vi "TEST - Conditional Auto-Indexing Tunnel.vi"(8 "error in (no error)":errorcluster) -> (0 "error out":errorcluster, 2 "Pass?":bool=TRUE)   [LabVIEW 2009]
doc: "This VI template can be used for the functional testing of VIs; this implementation includes handling for the testing of polymorphic VIs, and the polymorphic elements should be removed if not needed.\n\nCoded by Douglas A. Femec, January 24, 2006.\n\nCopyright (c) 2005-2006 MKS Instruments, Inc.\nAll rights reserved."
uses:
  TEST - Conditional Auto-Indexing Tunnel - Inputs.ctl
  Polymorphizer+ Data Type.ctl
  TEST - Conditional Auto-Indexing Tunnel - Outputs.ctl
  source/library/Conditional Auto-Indexing Tunnel/Conditional Auto-Indexing Tunnel (EXT).vi
  source/library/Conditional Auto-Indexing Tunnel/Conditional Auto-Indexing Tunnel (U64).vi
  source/library/Conditional Auto-Indexing Tunnel/Conditional Auto-Indexing Tunnel (I64).vi
  source/library/Conditional Auto-Indexing Tunnel/Conditional Auto-Indexing Tunnel (DBL).vi
  source/library/Conditional Auto-Indexing Tunnel/Conditional Auto-Indexing Tunnel (SGL).vi
  source/library/Conditional Auto-Indexing Tunnel/Conditional Auto-Indexing Tunnel (I32).vi
  source/library/Conditional Auto-Indexing Tunnel/Conditional Auto-Indexing Tunnel (I16).vi
  source/library/Conditional Auto-Indexing Tunnel/Conditional Auto-Indexing Tunnel (I8).vi
  source/library/Conditional Auto-Indexing Tunnel/Conditional Auto-Indexing Tunnel (U32).vi
  source/library/Conditional Auto-Indexing Tunnel/Conditional Auto-Indexing Tunnel (LVObject).vi
  source/library/Conditional Auto-Indexing Tunnel/Conditional Auto-Indexing Tunnel (U16).vi
  source/library/Conditional Auto-Indexing Tunnel/Conditional Auto-Indexing Tunnel (U8).vi
  source/library/Conditional Auto-Indexing Tunnel/Conditional Auto-Indexing Tunnel (CXT).vi
  source/library/Conditional Auto-Indexing Tunnel/Conditional Auto-Indexing Tunnel (CDB).vi
  source/library/Conditional Auto-Indexing Tunnel/Conditional Auto-Indexing Tunnel (CSG).vi
  source/library/Conditional Auto-Indexing Tunnel/Conditional Auto-Indexing Tunnel (Bool).vi
  source/library/Conditional Auto-Indexing Tunnel/Conditional Auto-Indexing Tunnel (String).vi
  source/library/Conditional Auto-Indexing Tunnel/Conditional Auto-Indexing Tunnel (Path).vi
  source/library/Conditional Auto-Indexing Tunnel/Conditional Auto-Indexing Tunnel (Variant).vi
  source/library/Conditional Auto-Indexing Tunnel/Conditional Auto-Indexing Tunnel (CTL-REF).vi
  source/library/Conditional Auto-Indexing Tunnel/Conditional Auto-Indexing Tunnel (GEN-REF).vi
  source/library/Conditional Auto-Indexing Tunnel/Conditional Auto-Indexing Tunnel (GObj-REF).vi
  source/library/Conditional Auto-Indexing Tunnel/Conditional Auto-Indexing Tunnel (VI-REF).vi
  TestClass/TestClass.lvclass
panel:
  in  "VI Refnum":refnum<vi>
  in  "GObj Refnum":refnum<vi>
  in  "Gen Refnum":refnum<vi>
  in  "Ctl Refnum":refnum<vi>
  out "Generated Outputs":T1[][](array[typedef]) {"Filtered Array Out" format="%.2f"}
  in  "Expected Outputs":T1[](array[typedef])=[{"Description"="Expect empty array", "Filtered Array Out"=[]}, {"Description"="Expect no elements kept", "Filtered Array Out"=[]}, {"Description"="Expect some elements kept", "Filtered Array Out"=[0.0, 0.0]}, {"Description"="Expect all elements kept", "Filtered Array Out"=[0.0, 1.0, 0.0, 1.0]}] {"Filtered Array Out" format="%.2f"}
  in  "Inputs":T2[](array[typedef])=[{"Description"="Empty arrays", "Data Types to Test"=[enum."EXT", enum."DBL", enum."SGL", enum."I32", enum."I16", enum."I8", enum."U32", enum."U16", enum."U8", enum."CXT", enum."CDB", enum."CSG", enum."Boolean", enum."String", enum."Path", enum."Variant", enum."CTL-REF", enum."GEN-REF", enum."GObj-REF", enum."VI-REF", enum."I64", enum."U64", enum."LabVIEW Object"], "Elements to keep"=[], "Array In"=[]}, {"Description"="No elements to keep", "Data Types to Test"=[enum."EXT", enum."DBL", enum."SGL", enum."I32", enum."I16", enum."I8", enum."U32", enum."U16", enum."U8", enum."CXT", enum."CDB", enum."CSG", enum."Boolean", enum."String", enum."Path", enum."Variant", enum."CTL-REF", enum."GEN-REF", enum."GObj-REF", enum."VI-REF", enum."I64", enum."U64", enum."LabVIEW Object"], "Elements to keep"=[FALSE, FALSE, FALSE, FALSE], "Array In"=[0.0, 0.0, 0.0, 0.0]}, {"Description"="Keep some elements", "Data Types to Test"=[enum."EXT", enum."DBL", enum."SGL", enum."I32", enum."I16", enum."I8", enum."U32", enum."U16", enum."U8", enum."CXT", enum."CDB", enum."CSG", enum."Boolean", enum."String", enum."Path", enum."Variant", enum."CTL-REF", enum."GEN-REF", enum."GObj-REF", enum."VI-REF", enum."I64", enum."U64", enum."LabVIEW Object"], "Elements to keep"=[TRUE, FALSE, TRUE, FALSE], "Array In"=[0.0, 1.0, 0.0, 1.0]}, {"Description"="Keep all elements", "Data Types to Test"=[enum."EXT", enum."DBL", enum."SGL", enum."I32", enum."I16", enum."I8", enum."U32", enum."U16", enum."U8", enum."CXT", enum."CDB", enum."CSG", enum."Boolean", enum."String", enum."Path", enum."Variant", enum."CTL-REF", enum."GEN-REF", enum."GObj-REF", enum."VI-REF", enum."I64", enum."U64", enum."LabVIEW Object"], "Elements to keep"=[TRUE, TRUE, TRUE, TRUE], "Array In"=[0.0, 1.0, 0.0, 1.0]}] {"Array In" format="%.2f"}
  # "Copyright (c) 2005-2006 MKS Instruments, Inc.\nAll rights reserved."
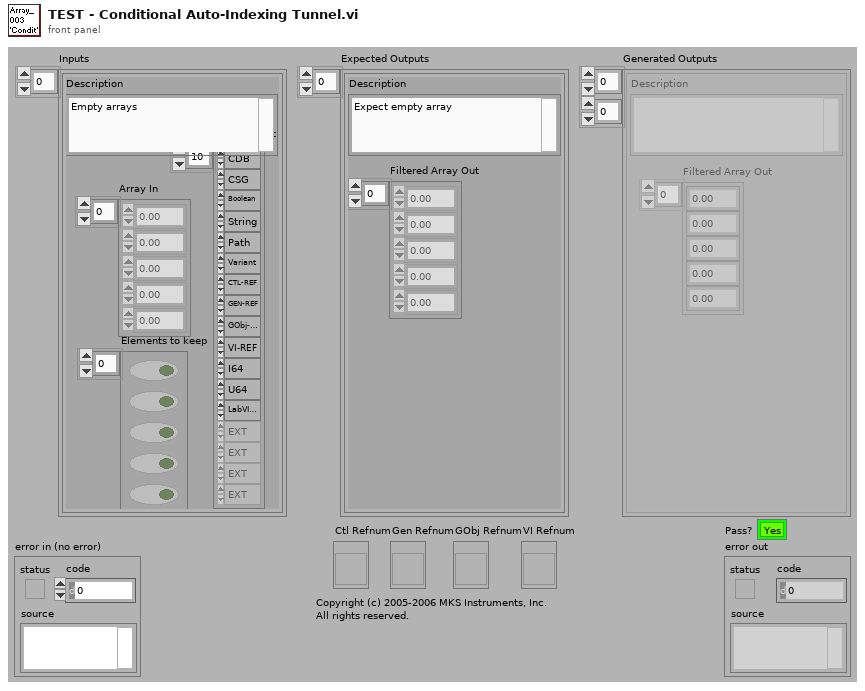
[diagram p1: front panel]
types:
  T1 = typedef "TEST - Conditional Auto-Indexing Tunnel - Outputs.ctl" = cluster{"Description":string, "Filtered Array Out":sgl[]}
  T2 = typedef "TEST - Conditional Auto-Indexing Tunnel - Inputs.ctl" = cluster{"Description":string, "Data Types to Test":T3[], "Elements to keep":bool[], "Array In":sgl[]}
  T3 = typedef "Polymorphizer+ Data Type.ctl" = enum16{"EXT", "DBL", "SGL", "I32", "I16", "I8", "U32", "U16", "U8", "CXT", "CDB", "CSG", "Boolean", "String", "Path", "Variant", "CTL-REF", "GEN-REF", "GObj-REF", "VI-REF", "ENUM", "ERR", "FILE-REF", "MENU-REF", "MENU-RING", "PICT-RING", "TXT&PICT-RING", "TXT-RING", "I64", "U64", "LabVIEW Object"}
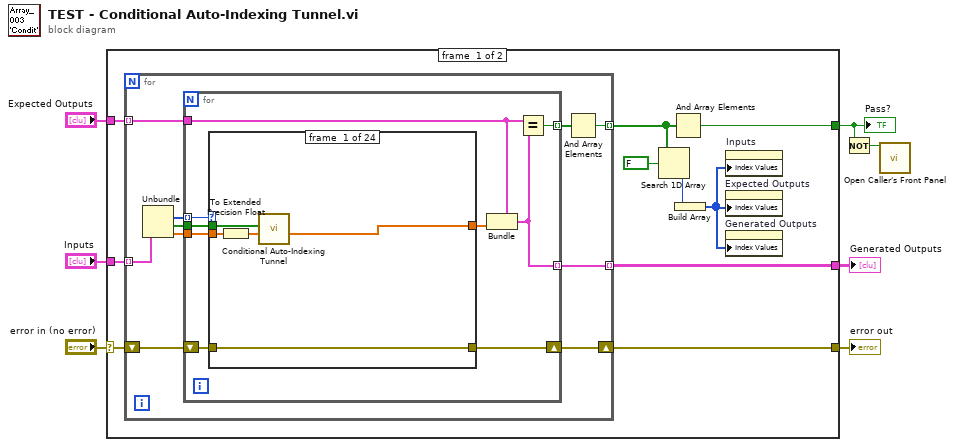
[diagram p0: block diagram]
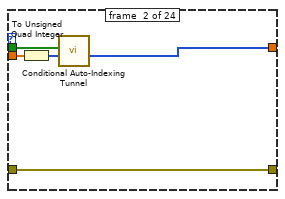
[diagram p2: hidden frame]
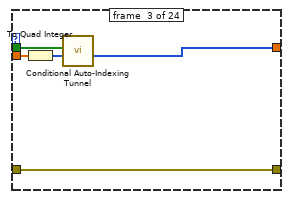
[diagram p3: hidden frame]
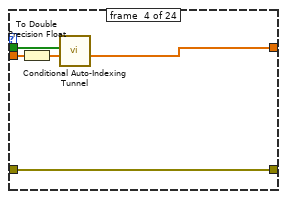
[diagram p4: hidden frame]
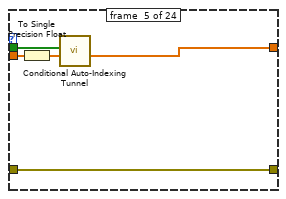
[diagram p5: hidden frame]
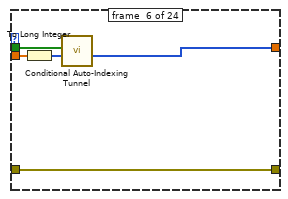
[diagram p6: hidden frame]
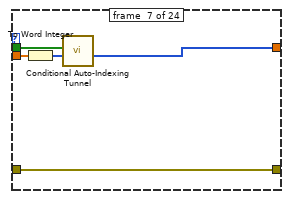
[diagram p7: hidden frame]
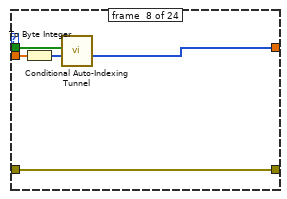
[diagram p8: hidden frame]
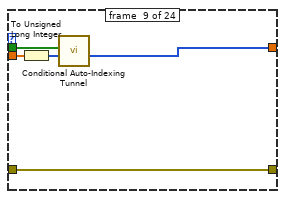
[diagram p9: hidden frame]
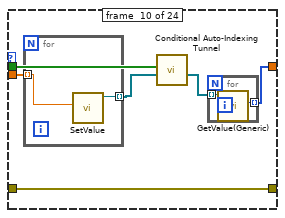
[diagram p10: hidden frame]
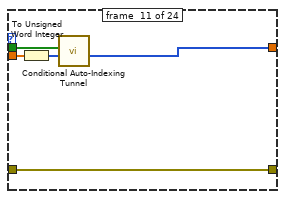
[diagram p11: hidden frame]
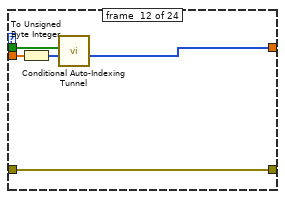
[diagram p12: hidden frame]
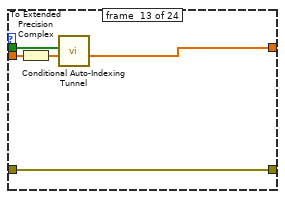
[diagram p13: hidden frame]
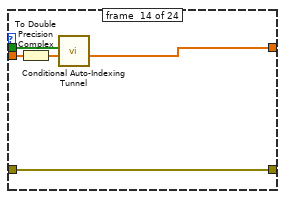
[diagram p14: hidden frame]
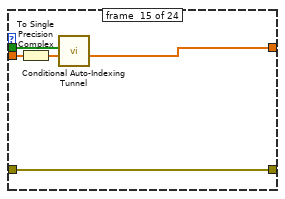
[diagram p15: hidden frame]
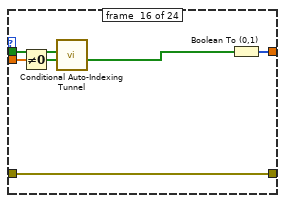
[diagram p16: hidden frame]
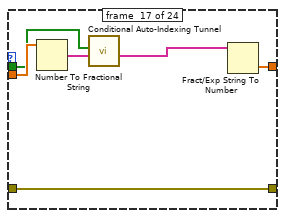
[diagram p17: hidden frame]
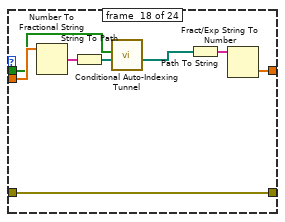
[diagram p18: hidden frame]
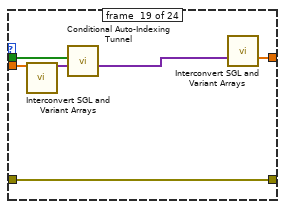
[diagram p19: hidden frame]
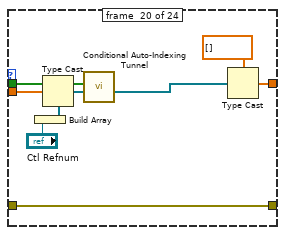
[diagram p20: hidden frame]
diagram:
  n1 = case shown="No Error" "error in (no error)" {
    selector: "error in (no error)" -> [w16 w181]
    tunnel: [w17 w181] -> w6
    tunnel: "Expected Outputs" -> [w14 _]
    tunnel: "Inputs" -> [w15 _]
    tunnel: [w13 _] -> w3
    tunnel: [w12 _] -> w1
    frame #0 {
      n2 = for {
        shift-right: [w22] -> w17
        shift-left: w16 -> [w23]
        tunnel: w15 -> [w24] mode=indexing
        tunnel: w14 -> [w27] mode=indexing
        tunnel: [w26] -> w13 mode=indexing
        tunnel: [w21] -> w11 mode=indexing
        n3 = Unbundle(w24) -> ("Data Types to Test"=w20:T3[], "Elements to keep"=w18:bool[], "Array In"=w19:sgl[])  [unwired: 1 out]
        n4 = for {
          tunnel: w27 -> [w36]
          tunnel: [w34] -> w26 mode=indexing
          tunnel: [w35] -> w25 mode=indexing
          shift-right: [w29] -> w22
          shift-left: w23 -> [w30]
          tunnel: w20 -> [w31] mode=indexing
          tunnel: w18 -> [w33]
          tunnel: w19 -> [w32]
          n5 = case shown="\"LabVIEW Object\"" w31 {
            tunnel: w33 -> [w37 w42 w47 w52 w57 w62 w67 w72 w77 w85 w92 w97 w102 w107 w112 w117 w123 w129 w141 w147 w156 w165 w174 _]
            tunnel: [w39 w44 w49 w54 w59 w64 w69 w74 w79 w82 w94 w99 w104 w109 w114 w121 w127 w134 w138 w146 w155 w164 w173 w180] -> w28
            tunnel: w32 -> [w41 w46 w51 w56 w61 w66 w71 w76 w81 w87 w96 w101 w106 w111 w116 w122 w128 w135 w140 w151 w160 w169 w178 w180]
            tunnel: w30 -> [w40 w45 w50 w55 w60 w65 w70 w75 w80 w86 w95 w100 w105 w110 w115 w120 w126 w132 w142 w150 w159 w168 w177 w179]
            tunnel: [w40 w45 w50 w55 w60 w65 w70 w75 w80 w86 w95 w100 w105 w110 w115 w120 w126 w132 w142 w150 w159 w168 w177 w179] -> w29
            frame #0 {
              n6 = To Extended Precision Float(1:w41) -> (0:w38:ext[])
              n7 = call-poly "Conditional Auto-Indexing Tunnel.vi"("Array in"=w38, "Elements to keep"=w37) -> ("Filtered Array out"=w39:ext[])  [unwired: 5 in]
            }
            frame #1 {
              n8 = To Unsigned Quad Integer(1:w46) -> (0:w43:u64[])
              n9 = call-poly "Conditional Auto-Indexing Tunnel.vi"("Array in"=w43, "Elements to keep"=w42) -> ("Filtered Array out"=w44:u64[])  [unwired: 5 in]
            }
            frame #2 {
              n10 = To Quad Integer(1:w51) -> (0:w48:i64[])
              n11 = call-poly "Conditional Auto-Indexing Tunnel.vi"("Array in"=w48, "Elements to keep"=w47) -> ("Filtered Array out"=w49:i64[])  [unwired: 5 in]
            }
            frame #3 {
              n12 = To Double Precision Float(number=w56) -> (double precision float=w53:dbl[])
              n13 = call-poly "Conditional Auto-Indexing Tunnel.vi"("Array in"=w53, "Elements to keep"=w52) -> ("Filtered Array out"=w54:dbl[])  [unwired: 5 in]
            }
            frame #4 {
              n14 = To Single Precision Float(number=w61) -> (single precision float=w58:sgl[])
              n15 = call-poly "Conditional Auto-Indexing Tunnel.vi"("Array in"=w58, "Elements to keep"=w57) -> ("Filtered Array out"=w59:sgl[])  [unwired: 5 in]
            }
            frame #5 {
              n16 = To Long Integer(number=w66) -> (32bit integer=w63:i32[])
              n17 = call-poly "Conditional Auto-Indexing Tunnel.vi"("Array in"=w63, "Elements to keep"=w62) -> ("Filtered Array out"=w64:i32[])  [unwired: 5 in]
            }
            frame #6 {
              n18 = To Word Integer(number=w71) -> (16bit integer=w68:i16[])
              n19 = call-poly "Conditional Auto-Indexing Tunnel.vi"("Array in"=w68, "Elements to keep"=w67) -> ("Filtered Array out"=w69:i16[])  [unwired: 5 in]
            }
            frame #7 {
              n20 = To Byte Integer(number=w76) -> (8bit integer=w73:i8[])
              n21 = call-poly "Conditional Auto-Indexing Tunnel.vi"("Array in"=w73, "Elements to keep"=w72) -> ("Filtered Array out"=w74:i8[])  [unwired: 5 in]
            }
            frame #8 {
              n22 = To Unsigned Long Integer(number=w81) -> (unsigned 32bit integer=w78:u32[])
              n23 = call-poly "Conditional Auto-Indexing Tunnel.vi"("Array in"=w78, "Elements to keep"=w77) -> ("Filtered Array out"=w79:u32[])  [unwired: 5 in]
            }
            frame #9 {
              n24 = for {
                tunnel: w87 -> [w91] mode=indexing
                tunnel: [w90] -> w84 mode=indexing
                n25 = call "SetValue.vi"("Value"=w91) -> ("TestClass out"=w90:refnum<class "TestClass.lvclass">)  [unwired: 9 in, 1 out]
              }
              n26 = call-poly "Conditional Auto-Indexing Tunnel.vi"("Array in"=w84, "Elements to keep"=w85) -> ("Filtered Array out"=w83:refnum<class>[])  [unwired: 5 in]
              n27 = for {
                tunnel: w83 -> [w89] mode=indexing
                tunnel: [w88] -> w82 mode=indexing
                n28 = call "GetValue(Generic).vi"("TestClass in"=w89) -> ("Value"=w88:i32)  [unwired: 8 in, 2 out]
              }
            }
            frame #10 {
              n29 = To Unsigned Word Integer(number=w96) -> (unsigned 16bit integer=w93:u16[])
              n30 = call-poly "Conditional Auto-Indexing Tunnel.vi"("Array in"=w93, "Elements to keep"=w92) -> ("Filtered Array out"=w94:u16[])  [unwired: 5 in]
            }
            frame #11 {
              n31 = To Unsigned Byte Integer(number=w101) -> (unsigned 8bit integer=w98:u8[])
              n32 = call-poly "Conditional Auto-Indexing Tunnel.vi"("Array in"=w98, "Elements to keep"=w97) -> ("Filtered Array out"=w99:u8[])  [unwired: 5 in]
            }
            frame #12 {
              n33 = To Extended Precision Complex(1:w106) -> (0:w103:cxt[])
              n34 = call-poly "Conditional Auto-Indexing Tunnel.vi"("Array in"=w103, "Elements to keep"=w102) -> ("Filtered Array out"=w104:cxt[])  [unwired: 5 in]
            }
            frame #13 {
              n35 = To Double Precision Complex(1:w111) -> (0:w108:cdb[])
              n36 = call-poly "Conditional Auto-Indexing Tunnel.vi"("Array in"=w108, "Elements to keep"=w107) -> ("Filtered Array out"=w109:cdb[])  [unwired: 5 in]
            }
            frame #14 {
              n37 = To Single Precision Complex(1:w116) -> (0:w113:csg[])
              n38 = call-poly "Conditional Auto-Indexing Tunnel.vi"("Array in"=w113, "Elements to keep"=w112) -> ("Filtered Array out"=w114:csg[])  [unwired: 5 in]
            }
            frame #15 {
              n39 = Not Equal To 0?(x=w122) -> (x != 0?=w118:bool[])
              n40 = call-poly "Conditional Auto-Indexing Tunnel.vi"("Array in"=w118, "Elements to keep"=w117) -> ("Filtered Array out"=w119:bool[])  [unwired: 5 in]
              n41 = Boolean To (0,1)(Boolean=w119) -> (0, 1=w121:i16[])
            }
            frame #16 {
              n42 = Number To Fractional String(number=w128) -> (F-format string=w124:string[])  [unwired: 3 in]
              n43 = call-poly "Conditional Auto-Indexing Tunnel.vi"("Array in"=w124, "Elements to keep"=w123) -> ("Filtered Array out"=w125:string[])  [unwired: 5 in]
              n44 = Fract/Exp String To Number(string=w125) -> (number=w127:dbl[])  [unwired: 3 in, 1 out]
            }
            frame #17 {
              n45 = Number To Fractional String(number=w135) -> (F-format string=w136:string[])  [unwired: 3 in]
              n46 = String To Path(string=w136) -> (path=w130:path[])
              n47 = call-poly "Conditional Auto-Indexing Tunnel.vi"("Array in"=w130, "Elements to keep"=w129) -> ("Filtered Array out"=w131:path[])  [unwired: 5 in]
              n48 = Path To String(path=w131) -> (string=w133:string[])
              n49 = Fract/Exp String To Number(string=w133) -> (number=w134:dbl[])  [unwired: 3 in, 1 out]
            }
            frame #18 {
              n50 = call "Interconvert SGL and Variant Arrays.vi"("SGL 1D Array In"=w140) -> ("Variant 1D Array Out"=w139:variant[])  [unwired: 10 in, 4 out]
              n51 = call-poly "Conditional Auto-Indexing Tunnel.vi"("Array in"=w139, "Elements to keep"=w141) -> ("Filtered Array out"=w137:variant[])  [unwired: 5 in]
              n52 = call "Interconvert SGL and Variant Arrays.vi"("Variant 1D Array In"=w137) -> ("SGL 1D Array Out"=w138:sgl[])  [unwired: 10 in, 4 out]
            }
            frame #19 {
              n53 = Build Array("Ctl Refnum") -> (w144:refnum<vi>[])
              n54 = Type Cast(type=w144, x=w151) -> (*(type *) &x=w148:refnum<vi>[])
              n55 = call-poly "Conditional Auto-Indexing Tunnel.vi"("Array in"=w148, "Elements to keep"=w147) -> ("Filtered Array out"=w149:refnum<vi>[])  [unwired: 5 in]
              n56 = Type Cast(type=sgl[] [], x=w149) -> (*(type *) &x=w146:sgl[])
            }
            frame #20 {
              n57 = Build Array("Gen Refnum") -> (w154:refnum<vi>[])
              n58 = Type Cast(type=w154, x=w160) -> (*(type *) &x=w157:refnum<vi>[])
              n59 = call-poly "Conditional Auto-Indexing Tunnel.vi"("Array in"=w157, "Elements to keep"=w156) -> ("Filtered Array out"=w158:refnum<vi>[])  [unwired: 5 in]
              n60 = Type Cast(type=sgl[] [], x=w158) -> (*(type *) &x=w155:sgl[])
            }
            frame #21 {
              n61 = Build Array("GObj Refnum") -> (w163:refnum<vi>[])
              n62 = Type Cast(type=w163, x=w169) -> (*(type *) &x=w166:refnum<vi>[])
              n63 = call-poly "Conditional Auto-Indexing Tunnel.vi"("Array in"=w166, "Elements to keep"=w165) -> ("Filtered Array out"=w167:refnum<vi>[])  [unwired: 5 in]
              n64 = Type Cast(type=sgl[] [], x=w167) -> (*(type *) &x=w164:sgl[])
            }
            frame #22 {
              n65 = Build Array("VI Refnum") -> (w172:refnum<vi>[])
              n66 = Type Cast(type=w172, x=w178) -> (*(type *) &x=w175:refnum<vi>[])
              n67 = call-poly "Conditional Auto-Indexing Tunnel.vi"("Array in"=w175, "Elements to keep"=w174) -> ("Filtered Array out"=w176:refnum<vi>[])  [unwired: 5 in]
              n68 = Type Cast(type=sgl[] [], x=w176) -> (*(type *) &x=w173:sgl[])
            }
            frame #23 {
            }
          }
          n69 = Bundle(cluster=w36, "Filtered Array Out"=w28) -> (w34:T1)  [unwired: 1 in]
          n70 = Equal?(x=w36, y=w34) -> (x = y?=w35:bool)
        }
        n71 = And Array Elements(Boolean array=w25) -> (logical AND=w21:bool)
      }
      n72 = Search 1D Array(1D array=w11, element=FALSE) -> (index of element=w9:i32)  [unwired: 1 in]
      n73 = And Array Elements(Boolean array=w11) -> (logical AND=w12:bool)
      n74 = Build Array(w9) -> (w8:i32[])
      n75 = property on="Inputs" class="Arr (strict)"("Index Values"=w8) -> ()  [unwired: 2 in, 2 out]
      n76 = property on="Expected Outputs" class="Arr (strict)"("Index Values"=w8) -> ()  [unwired: 2 in, 2 out]
      n77 = property on="Generated Outputs" class="Arr (strict)"("Index Values"=w8) -> ()  [unwired: 2 in, 2 out]
    }
    frame #1 {
    }
  }
  "error out" <- w6
  "Pass?" <- w1
  "Generated Outputs" <- w3
  n78 = Not(x=w1) -> (.not. x?=w2:bool)
  n79 = call "Open Caller's Front Panel.vi"("Open?"=w2) -> ()  [unwired: 14 in, 1 out]
